vi "pruebas_rgb.vi"() -> ()   [LabVIEW 2025]
panel:
  out "read buffer":string
  in  "Color Box":u32(colorbox)
  out "error out":errorcluster
  in  "VISA resource name":refnum<visa-resource-name>
  in  "stop":bool
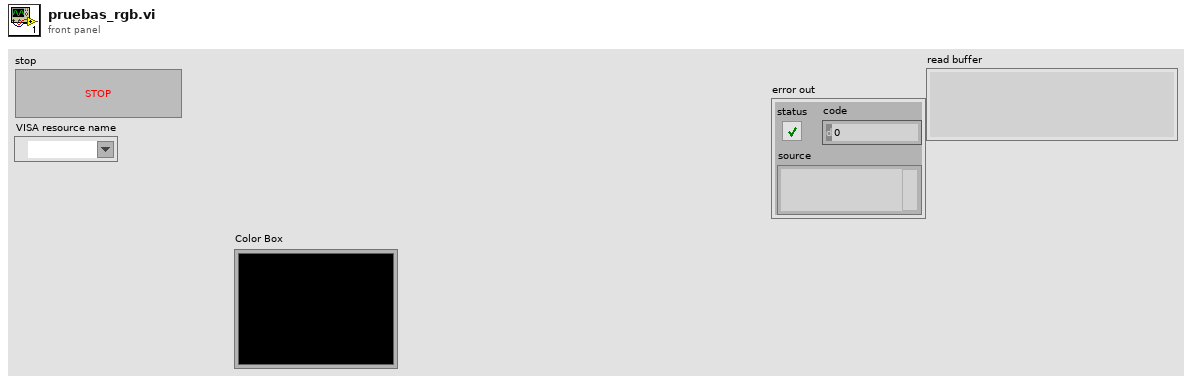
[diagram p1: front panel]
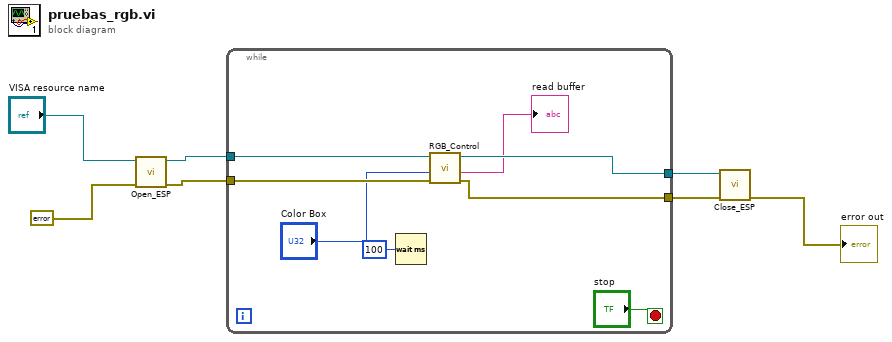
[diagram p0: block diagram]
diagram:
  n1 = call "Open_ESP.vi"("error in (no error)"=errorcluster {"status"=FALSE, "code"=0, "source"=""}, "VISA resource name"="VISA resource name") -> ("error out"=w6:errorcluster, "VISA resource name out"=w7:refnum<visa-resource-name>)  [unwired: 8 in]
  n2 = while {
    tunnel: w7 -> [w14]
    tunnel: w6 -> [w13]
    tunnel: [w12] -> w5
    tunnel: [w11] -> w4
    stop <- "stop" stop-if-true
    n3 = Wait (ms)(milliseconds to wait=u32 100) -> ()  [unwired: 1 out]
    n4 = call "RGB_Control.vi"("error in (no error)"=w13, "Color Box"="Color Box", "VISA resource name"=w14) -> ("error out"=w12:errorcluster, "read buffer"=→"read buffer":string, "VISA resource name out"=w11:refnum<visa-resource-name>)  [unwired: 6 in]
  }
  n5 = call "Close_ESP.vi"("error in (no error)"=w5, "VISA resource name"=w4) -> ("error out"=→"error out":errorcluster)  [unwired: 9 in]
